vi "Get AO Res.vi"(8 "Error In":errorcluster, 11 "LINX Device Config":T1) -> (0 "Error Out":errorcluster, 2 "AO Res":u8, 3 "LINX Device Config":T1)   [LabVIEW 2019, in "LINXx.lvlib"]
uses:
  <vilib>/MakerHub/LINX/Private/Device/Type Defs/LINX Device Config.ctl
  <vilib>/MakerHub/LINX/Private/Type Defs/Interface.ctl
  <vilib>/MakerHub/LINX/Private/Device/Type Defs/TCP Config.ctl
  <vilib>/MakerHub/LINX/Private/Device/Type Defs/Channels.ctl
  <vilib>/MakerHub/LINX/Private/Type Defs/Error Type.ctl
  LINXx.lvlib
  <vilib>/MakerHub/LINX/Private/Device/Device.lvlib
  <vilib>/MakerHub/LINX/LMH-LINX.lvlib
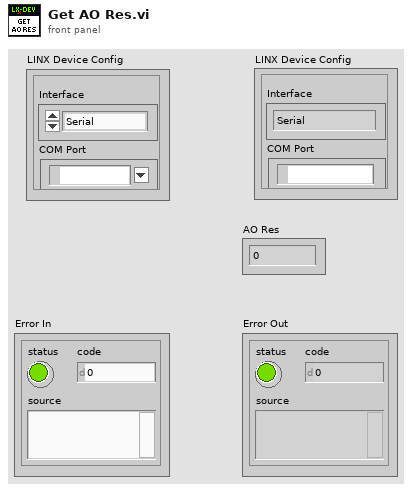
[diagram p1: front panel]
types:
  T1 = typedef "LMH-LINX.lvlib/Device.lvlib/LINX Device Config.ctl" = cluster{"Interface":T2, "COM Port":refnum<visa-resource-name>, "TCP Configuration":T3, "Device Family":u8, "Device ID":u8, "Device Name":string, "TCP Ref":refnum<k5>, "Channels":T4}
  T2 = typedef "LMH-LINX.lvlib/Interface.ctl" = enum16{"Serial", "TCP"}
  T3 = typedef "LMH-LINX.lvlib/Device.lvlib/TCP Config.ctl" = cluster{"IP Address":string, "Port":u16}
  T4 = typedef "LMH-LINX.lvlib/Channels.ctl" = cluster{"DI":u8[], "DO":u8[], "AI":u8[], "AO":u8[], "PWM":u8[], "QE":u8[], "UART":u8[], "I2C 2":u8[], "SPI":u8[], "CAN":u8[], "Servo":u8[], "AI Ref (V)":dbl, "AI Resolution (Bits)":u8, "AO Ref (V)":dbl, "AO Resolution (Bits)":u8}
  T5 = typedef "LMH-LINX.lvlib/Error Type.ctl" = enum16{"Unknown", "Timeout", "Corrupt Return Packet", "Unable To Connect", "Command Not Supported", "Channel DNE", "Invalid COM Config", "Firmware Version Mismatch", "myRIO Support", "CMD Specific Error", "Local IO Not Supported"}
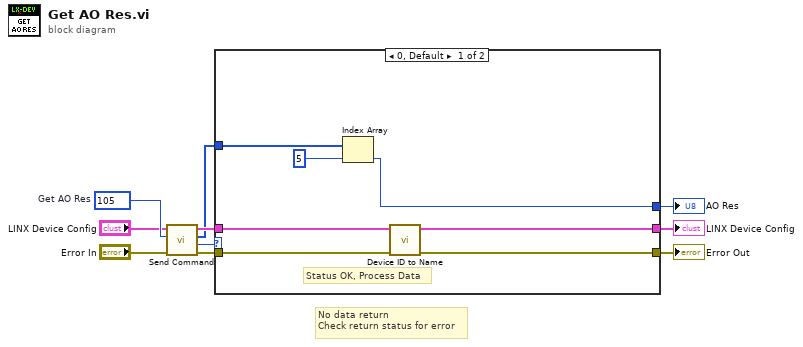
[diagram p0: block diagram]
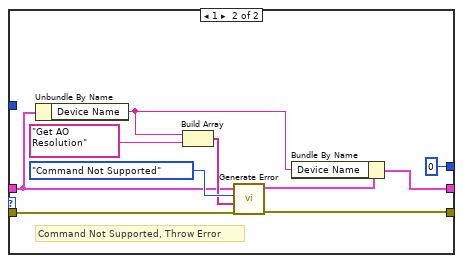
[diagram p2: hidden frame]
diagram:
  w9 = u16 105  # Get AO Res
  # "No data return\nCheck return status for error"
  n1 = call <vilib>:"Send Command.vi"("Error In"="Error In", "CMD"=w9, "LINX Device Config"="LINX Device Config") -> ("Error Out"=w4:errorcluster, "Status"=w2:u8, "Response"=w3:u8[], "LINX Device Config"=w6:T1)  [unwired: 5 in]
  n2 = case shown="0, Default" w2 {
    tunnel: [w14 w21] -> w7
    tunnel: w6 -> [w17 w20]
    tunnel: [w15 w26] -> w5
    tunnel: w4 -> [w16 w27]
    tunnel: w3 -> [w13 _]
    tunnel: [w11 u8 0] -> w1
    frame 0, Default {
      # "Status OK, Process Data"
      n3 = Index Array(array=w13, index=5) -> (element=w11:u8)
      n4 = call <vilib>:"Device ID to Name.vi"("Error In"=w16, "LINX Device Config"=w17) -> ("Error Out"=w15:errorcluster, "LINX Device Config"=w14:T1)  [unwired: 7 in, 1 out]
    }
    frame 1 {
      # "Command Not Supported, Throw Error"
      n5 = Unbundle By Name(w20) -> ("Device Name"=w19:string)
      n6 = Build Array(w19, "Get AO Resolution") -> (w23:string[])
      n7 = call <vilib>:"Generate Error.vi"("Error In"=w27, "Arguments"=w23, "Error Type"=Error_Type."Command Not Supported", "LINX Device Config"=w20) -> ("Error Out"=w26:errorcluster, "Dup LINX Device Config"=w22:T1)  [unwired: 6 in]
      n8 = Bundle By Name(cluster=w22, "Device Name"=w19) -> (w21:T1)
    }
  }
  "Error Out" <- w5
  "LINX Device Config" <- w7
  "AO Res" <- w1
